vi "getTaskInfos.vi"(8 "error in (no error)":errorcluster, 11 "BuildServer in":refnum<class "BuildServer.lvclass">) -> (0 "error out":errorcluster, 3 "BuildServer out":refnum<class "BuildServer.lvclass">)   [LabVIEW 2017, in "BuildServer.lvlib" / "BuildServer.lvclass"]
uses:
  BuildServer.lvclass
  <vilib>/Ekim/LUT/LUT/LUT.lvclass
  BuildWorker/Classes/Task/Task.lvclass
panel:
  out "Project Name":string[][](array[string])
  out "BuildSpec Name":string[][](array[string])
  out "BuildSpec Type":string[][](array[string])
  out "Target":string[][](array[string])
  out "Task Name":string[][](array[string])
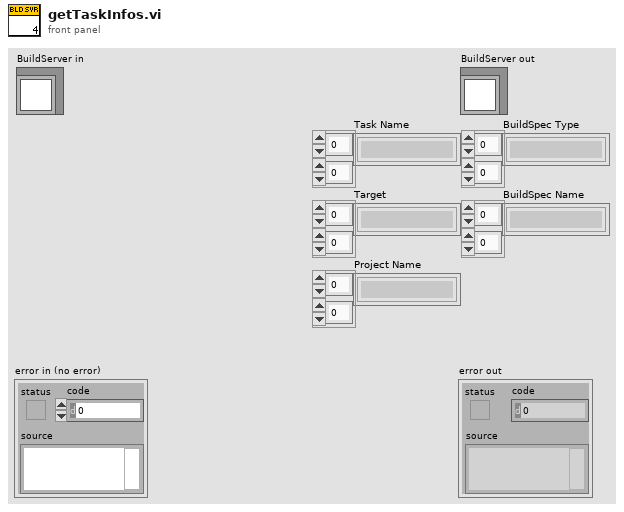
[diagram p1: front panel]
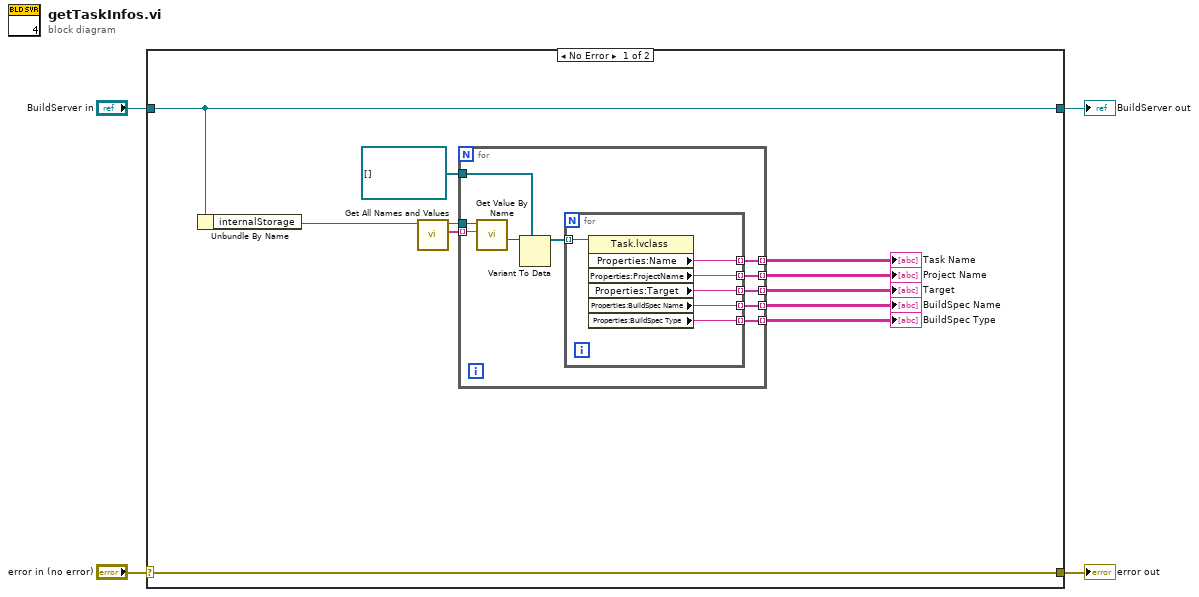
[diagram p0: block diagram]
diagram:
  n1 = case shown="No Error" "error in (no error)" {
    selector: "error in (no error)" -> [w15 w33]
    tunnel: [w15 w33] -> w3
    tunnel: [w14 w32] -> w1
    tunnel: "BuildServer in" -> [w14 w32]
    frame No Error {
      n2 = Unbundle By Name(w14) -> ("internalStorage"=w13:refnum<class "LUT.lvclass">)
      n3 = call <vilib>:"Get All Names and Values.vi"("LUT in"=w13) -> ("Names"=w5:string[], "LUT out"=w12:refnum<class "LUT.lvclass">)  [unwired: 7 in, 2 out]
      n4 = for {
        tunnel: refnum<class "Task.lvclass">[] [] -> [w22]
        tunnel: w12 -> [w25]
        tunnel: w5 -> [w24] mode=indexing
        tunnel: [w20] -> w10 mode=indexing
        tunnel: [w19] -> w9 mode=indexing
        tunnel: [w18] -> w8 mode=indexing
        tunnel: [w17] -> w7 mode=indexing
        tunnel: [w16] -> w6 mode=indexing
        n5 = call <vilib>:"Get Value By Name.vi"("Name"=w24, "LUT in"=w25) -> ("Value"=w23:variant)  [unwired: 6 in, 3 out]
        n6 = Variant To Data(type=w22, Variant=w23) -> (data=w21:refnum<class "Task.lvclass">[])  [unwired: 1 in, 1 out]
        n7 = for {
          tunnel: w21 -> [w31] mode=indexing
          tunnel: [w30] -> w20 mode=indexing
          tunnel: [w29] -> w19 mode=indexing
          tunnel: [w28] -> w18 mode=indexing
          tunnel: [w27] -> w17 mode=indexing
          tunnel: [w26] -> w16 mode=indexing
          n8 = property class="Task.lvclass"(reference=w31) -> ("Properties:Name"=w30:string, "Properties:ProjectName"=w29:string, "Properties:Target"=w28:string, "Properties:BuildSpec Name"=w27:string, "Properties:BuildSpec Type"=w26:string)  [unwired: 1 in, 2 out]
        }
      }
      "Task Name" <- w10
      "Target" <- w8
      "BuildSpec Type" <- w6
      "BuildSpec Name" <- w7
      "Project Name" <- w9
    }
    frame Error {
    }
  }
  "error out" <- w3
  "BuildServer out" <- w1
